vi "Create.vi"(5 "Is Greater Than in":refnum<class "Is Greater Than.lvclass">, 8 "error in (no error)":errorcluster, 11 "Expected":variant) -> (0 "error out":errorcluster, 3 "Is Greater Than":refnum<class "Is Greater Than.lvclass">)   [LabVIEW 2017, in "Transparent Assertions.lvlib" / "Is Greater Than.lvclass"]
uses:
  Is Greater Than.lvclass
  Is Greater Than.lvclass/Is Greater Than.ctl
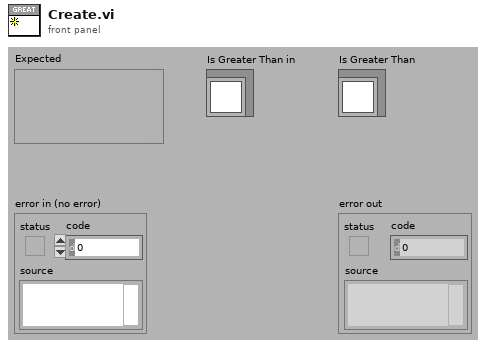
[diagram p1: front panel]
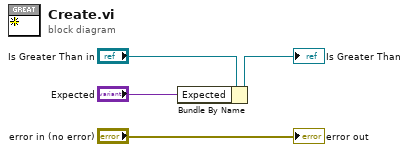
[diagram p0: block diagram]
diagram:
  n1 = Bundle By Name(cluster="Is Greater Than in", "Expected"="Expected") -> (→"Is Greater Than":refnum<class "Is Greater Than.lvclass">)
  "error out" <- "error in (no error)"
